vi "Power Accuracy Find Pad Values.vi"(11 "Test Parameters":T1={"Stimulus"={"Power Start"=0, "Power Stop"=44, "Frequency Type"=enum."Band Edges", "Frequency Points"=[], "TX 1 Frequency (MHz)"={"Min"=0.0, "Max"=0.0}, "TX 2 Frequency (MHz)"={"Min"=0.0, "Max"=0.0}, "RX Frequency (MHz)"={"Min"=0.0, "Max"=0.0}, "Pad Model Number"="", "Pad Serial Number"="", "Pad Values"=[]}, "Measurement"={"DUT Port"=enum."Port 1", "Direction"=0}, "Display"={"Power"={"Min"=-1, "Max"=-1}, "Tolerance"={"Min"=-1.0, "Max"=-1.0}}, "Limit"={"Tolerance"=44.0}, "Calibration"={"Calibrated?"=FALSE}} {"Measurement"."Direction" items=["Reverse", "Forward", "Auxiliary"]}) -> (2 "Values Present?":bool, 3 "Pad Values Out":dbl[][](array[numeric]))   [LabVIEW 2011]
uses:
  TypeDefs/Power Accuracy Test Parameters.ctl
  TypeDefs/Power Accuracy Stimulus Parameters.ctl
  TypeDefs/Power Accuracy Measurement Parameters.ctl
  SI.LIB/PIM.LIB/HW IO/DUTport.ctl
  SI.LIB/PIM.LIB/HW IO/MeasMode.ctl
  TypeDefs/Power Accuracy Display Parameters.ctl
  TypeDefs/Power Accuracy Limit Parameters.ctl
  TypeDefs/Power Accuracy Calibration State.ctl
  OpenG.LIB/array/array.llb/Filter 1D Array with Scalar (DBL)__ogtk.vi
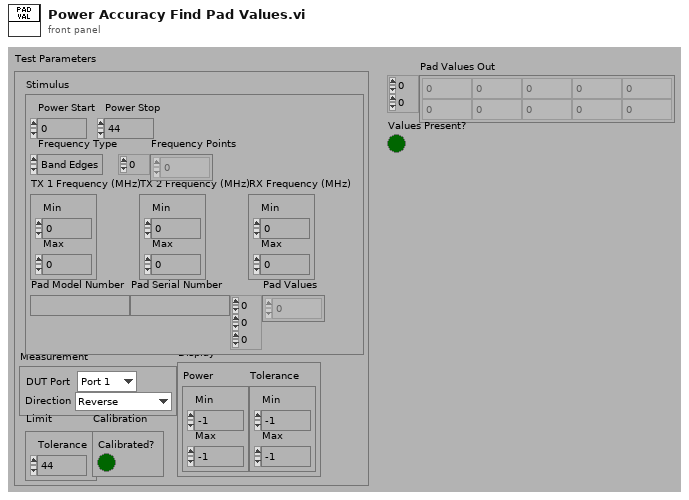
[diagram p1: front panel]
types:
  T1 = typedef "Power Accuracy Test Parameters.ctl" = cluster{"Stimulus":T2, "Measurement":T3, "Display":T6, "Limit":T7, "Calibration":T8}
  T2 = typedef "Power Accuracy Stimulus Parameters.ctl" = cluster{"Power Start":i32, "Power Stop":i32, "Frequency Type":enum16{"Band Edges", "Custom"}, "Frequency Points":dbl[], "TX 1 Frequency (MHz)":cluster{"Min":dbl, "Max":dbl}, "TX 2 Frequency (MHz)":cluster{"Min":dbl, "Max":dbl}, "RX Frequency (MHz)":cluster{"Min":dbl, "Max":dbl}, "Pad Model Number":string, "Pad Serial Number":string, "Pad Values":dbl[][][]}
  T3 = typedef "Power Accuracy Measurement Parameters.ctl" = cluster{"DUT Port":T4, "Direction":T5}
  T4 = typedef "DUTport.ctl" = enum16{"Port 1", "Port 2"}
  T5 = typedef "MeasMode.ctl" = u16
  T6 = typedef "Power Accuracy Display Parameters.ctl" = cluster{"Power":cluster{"Min":i32, "Max":i32}, "Tolerance":cluster{"Min":dbl, "Max":dbl}}
  T7 = typedef "Power Accuracy Limit Parameters.ctl" = cluster{"Tolerance":dbl}
  T8 = typedef "Power Accuracy Calibration State.ctl" = cluster{"Calibrated?":bool}
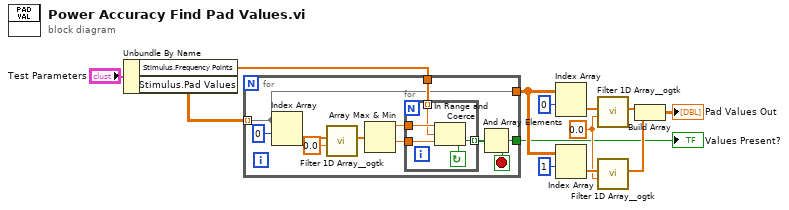
[diagram p0: block diagram]
diagram:
  w5 = 0.0
  n1 = Unbundle By Name("Test Parameters") -> ("Stimulus.Frequency Points"=w13:dbl[], "Stimulus.Pad Values"=w12:dbl[][][])
  n2 = for {
    tunnel: w12 -> [w14] mode=indexing
    tunnel: w13 -> [w22]
    tunnel: [w20] -> w2
    tunnel: [w14] -> w4
    stop <- w20 stop-if-true
    n3 = Index Array(array=w14, index (row)=0 ("disabled index (col)")) -> (element=w15:dbl[])  [unwired: 1 in]
    n4 = call-poly "Filter 1D Array__ogtk.vi"("items to filter"=0.0, "array"=w15) -> ("filtered array"=w16:dbl[])  [unwired: 4 in, 1 out]
    n5 = Array Max & Min(array=w16) -> (max value=w19:dbl, min value=w18:dbl)  [unwired: 2 out]
    n6 = for {
      tunnel: w22 -> [w25] mode=indexing
      tunnel: w19 -> [w27]
      tunnel: w18 -> [w26]
      tunnel: [w24] -> w21 mode=indexing
      stop <- w24 continue-if-true
      n7 = In Range and Coerce(upper limit=w27, x=w25, lower limit=w26) -> (In Range?=w24:bool)  [unwired: 1 out]
    }
    n8 = And Array Elements(Boolean array=w21) -> (logical AND=w20:bool)
  }
  "Values Present?" <- w2
  n9 = Index Array(array=w4, index (row)=0 ("disabled index (col)")) -> (element=w11:dbl[])  [unwired: 1 in]
  n10 = Index Array(array=w4, index (row)=1 ("disabled index (col)")) -> (element=w8:dbl[])  [unwired: 1 in]
  n11 = call-poly "Filter 1D Array__ogtk.vi"("items to filter"=w5, "array"=w11) -> ("filtered array"=w7:dbl[])  [unwired: 4 in, 1 out]
  n12 = call-poly "Filter 1D Array__ogtk.vi"("items to filter"=w5, "array"=w8) -> ("filtered array"=w6:dbl[])  [unwired: 4 in, 1 out]
  n13 = Build Array(w7, w6) -> (→"Pad Values Out":dbl[][])
